vi "CheckingSerialPortStatus.vi"(9 "error in":errorcluster, 10 "Baud":i16(ring)=-1 items=["Unknown"=-1, "Unasserted"=0, "Asserted"=1], 11 "VISA  name":refnum<visa-resource-name>) -> (3 "error output":errorcluster)   [LabVIEW 2023]
panel:
  in  "BreakState":i16(ring)=-1 items=["Unknown"=-1, "Unasserted"=0, "Asserted"=1]
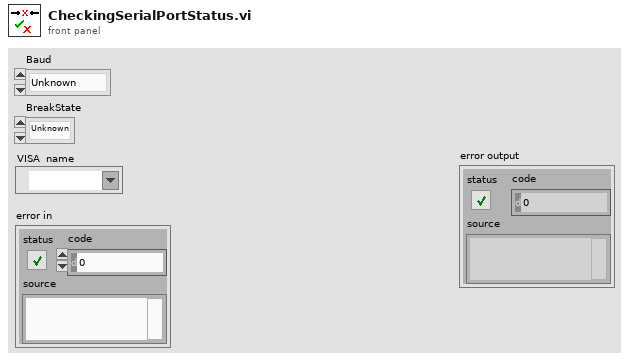
[diagram p1: front panel]
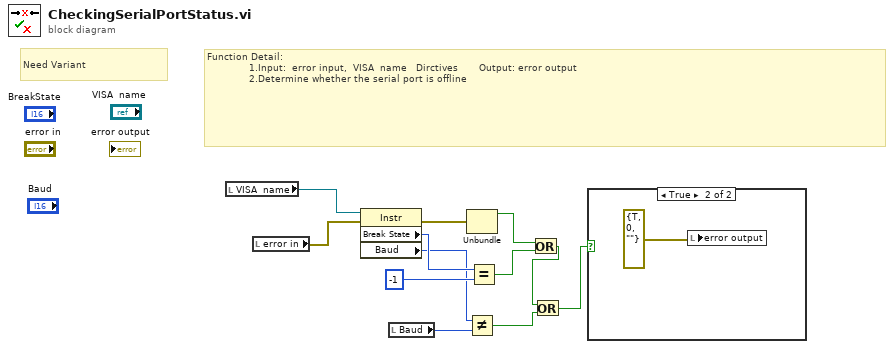
[diagram p0: block diagram]
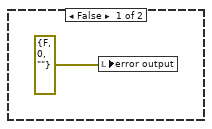
[diagram p2: hidden frame]
diagram:
  # "Need Variant"
  # "Function Detail:\n              1.Input:  error input,  VISA  name   Dirctives       Output: error output\n              2.Determine whether the serial port is offline"
  n1 = local read "VISA  name"() -> (w11:refnum<visa-resource-name>)
  n2 = local read "error in"() -> (w12:errorcluster)
  n3 = property class="Instr"(reference=w11, error in=w12) -> (error out=w8:errorcluster, "Break State"=w9:i16, "Baud"=w5:u32)  [unwired: 1 out]
  n4 = local read "Baud"() -> (w4:i16)
  n5 = Unbundle(w8) -> ("status"=w7:bool)  [unwired: 2 out]
  n6 = Not Equal?(x=w5, y=w4) -> (x != y?=w2:bool)
  n7 = Equal?(x=w9, y=i16 -1) -> (x = y?=w6:bool)
  n8 = Or(x=w7, y=w6) -> (x .or. y?=w3:bool)
  n9 = Or(x=w3, y=w2) -> (x .or. y?=w1:bool)
  n10 = case shown="True" w1 {
    frame False {
      n11 = local write "error output"(errorcluster {"status"=FALSE, "code"=0, "source"=""} ("error output (no error)")) -> ()
    }
    frame True {
      n12 = local write "error output"(errorcluster {"status"=TRUE, "code"=0, "source"=""} ("error output (no error)")) -> ()
    }
  }
